vi "trigger_rising_edge_diag.vi"(10 "Ref_MLD measurement":dbl[][](array[numeric]), 11 "dt in":dbl) -> (3 "Waveform":waveform(dbl), 4 "First Rising edge index":i32, 6 "Frequency":dbl, 7 "Ref_MLD_triggered":dbl[][](array[numeric]))   [LabVIEW 2013]
uses:
  <vilib>/Analysis/baseanly.llb/Mean (DBL).vi
  <vilib>/Analysis/NI_AALBase.lvlib
panel:
  out "Waveform Graph 3":dbl[](graph)
  out "Waveform Graph 2":dbl[](graph)
  out "Waveform Graph":waveform(dbl)(graph)
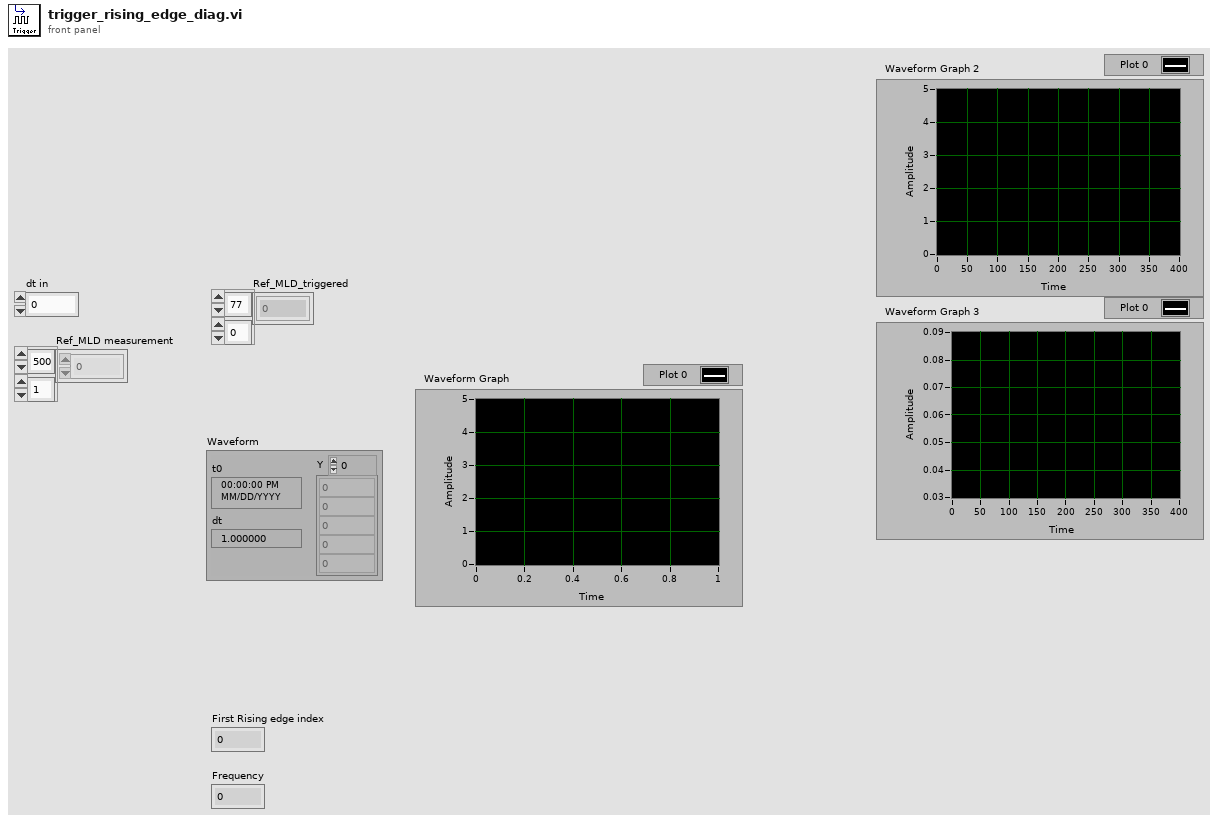
[diagram p1: front panel]
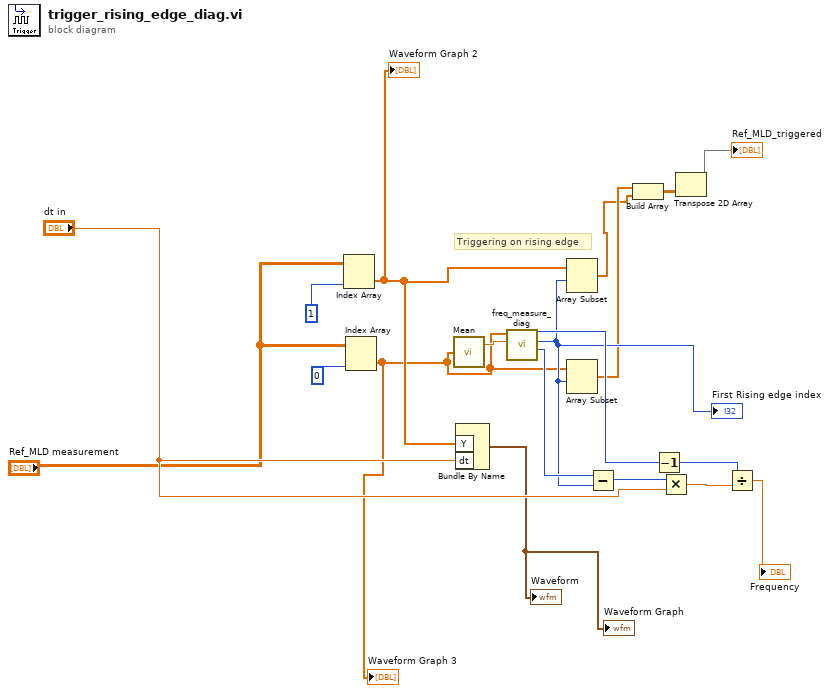
[diagram p0: block diagram]
diagram:
  # "Triggering on rising edge"
  n1 = Index Array(array="Ref_MLD measurement", index (col)=1 ("index (row)")) -> (element=w4:dbl[])  [unwired: 1 in]
  "Waveform Graph 2" <- w4
  n2 = Index Array(array="Ref_MLD measurement", index (col)=0 ("index (row)")) -> (element=w3:dbl[])  [unwired: 1 in]
  "Waveform Graph 3" <- w3
  n3 = call-poly <vilib>:"Mean.vi"("X"=w3) -> ("mean"=w15:dbl)  [unwired: 1 out]
  n4 = Bundle By Name("Y"=w4, "dt"="dt in") -> (→"Waveform" →"Waveform Graph":waveform(dbl))  [unwired: 1 in]
  n5 = call "freq_measure_diag.vi"("Ref_average"=w15, "data"=w3) -> ("Actual (last) Rising edge index"=w12:i32, "First Rising edge index"=w5:i32, "Rising edges"=w9:i32)  [unwired: 7 in]
  "First Rising edge index" <- w5
  n6 = Array Subset(array=w4, index=w5) -> (w1:dbl[])  [unwired: 1 in]
  n7 = Array Subset(array=w3, index=w5) -> (w2:dbl[])  [unwired: 1 in]
  n8 = Subtract(x=w12, y=w5) -> (x-y=w14:i32)
  n9 = Build Array(w2, w1) -> (w18:dbl[][])
  n10 = Decrement(x=w9) -> (x-1=w8:i32)
  n11 = Multiply(x=w14, y="dt in") -> (x*y=w13:dbl)
  n12 = Transpose 2D Array(2D array=w18) -> (transposed array=→"Ref_MLD_triggered":dbl[][])
  n13 = Divide(x=w8, y=w13) -> (x/y=→"Frequency":dbl)
